vi "GV_StoreNewZoomValue.vi"(7 "Immediate":bool, 8 "error in (no error)":errorcluster, 11 "Gviewer in":refnum<class "Gviewer.lvclass">) -> (0 "error out":errorcluster, 3 "Gviewer out":refnum<class "Gviewer.lvclass">)   [LabVIEW 2020, in "Sgraph_lib_V1.lvlib" / "Gviewer.lvclass"]
doc: "Set the new pan or zoom value to the undo memory"
uses:
  Gviewer.lvclass
  Gviewer.lvclass/Gviewer.ctl
  controls/Typedef_ZoomEvent.ctl
  controls/Typedef_Live.ctl
  controls/Typedef_SelProperties.ctl
  controls/Typedef_LineType.ctl
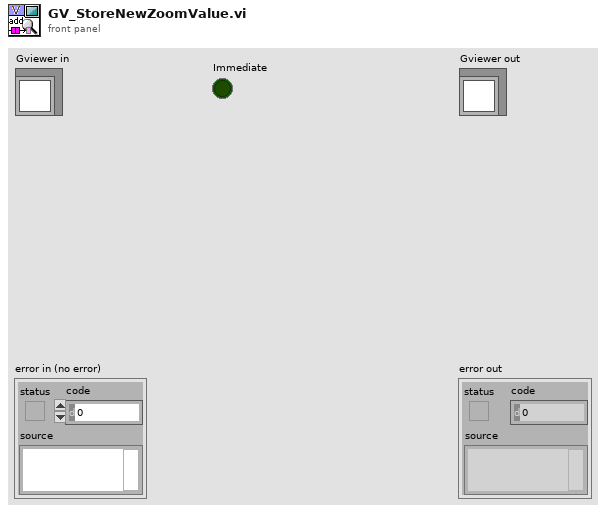
[diagram p1: front panel]
types:
  T1 = typedef "Sgraph_lib_V1.lvlib/Gviewer.lvclass/Typedef_ZoomEvent.ctl" = cluster{"Time-Start":timestamp, "Time-End":timestamp, "TimeSpan(sec)":dbl, "Live":T2, "SelProperties":T3[], "Time Stamp":timestamp}
  T2 = typedef "Sgraph_lib_V1.lvlib/Gviewer.lvclass/Typedef_Live.ctl" = enum16{"Live View", "Freeze"}
  T3 = typedef "Sgraph_lib_V1.lvlib/Gviewer.lvclass/Typedef_SelProperties.ctl" = cluster{"Color":u32, "LineType":T4, "max":dbl, "min":dbl}
  T4 = typedef "Sgraph_lib_V1.lvlib/Gviewer.lvclass/Typedef_LineType.ctl" = enum16{"num_bare", "num_MinMax_Area", "num_MinMax_Lines", "num_MinMax_Forfor", "num_Max_Area", "num_Max_Line", "num_Max_Forfor", "num_Min_Area", "num_Min_Line", "num_Min_Fosfor", "Boolean_Line_01", "Boolean_Area_01", "Boolean_Fosfor_01", "Boolean_Line_TF", "Boolean_Area_TF", "Boolean_Fosfor_TF", "Boolean_OnOff_Line", "Boolean_OnOff_Area", "Boolean_OnOff_Fosfor", "Boolean_spare", "StringEvent_Line", "StringEvent_TimeLine"}
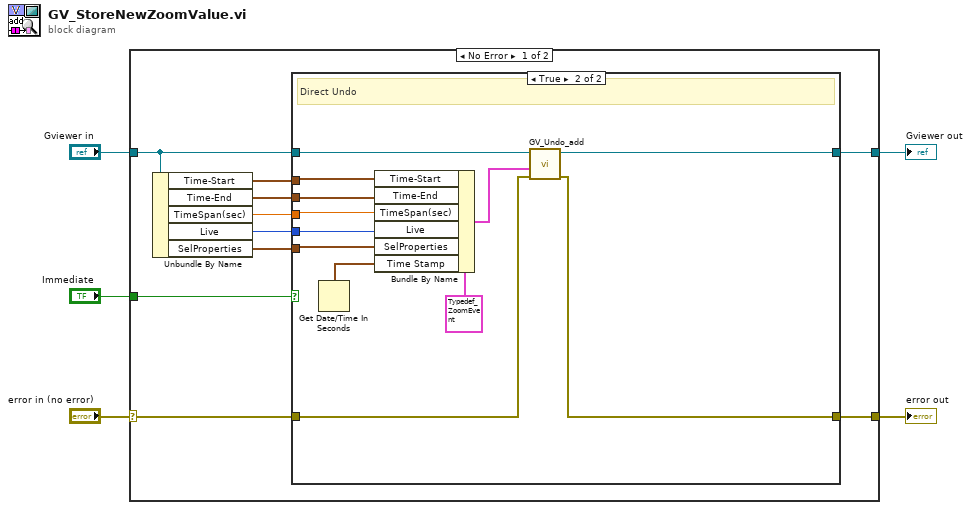
[diagram p0: block diagram]
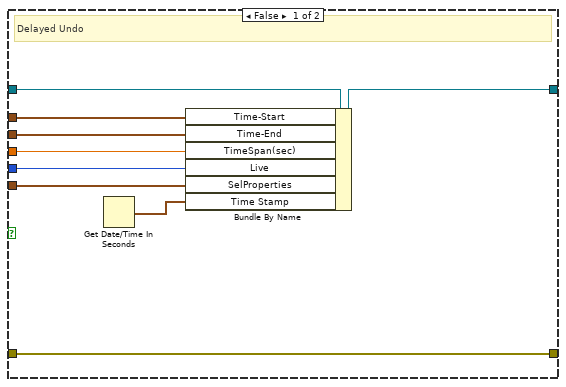
[diagram p2: hidden frame]
diagram:
  n1 = case shown="No Error" "error in (no error)" {
    selector: "error in (no error)" -> [w8 w38]
    tunnel: [w6 w38] -> w4
    tunnel: [w7 w37] -> w2
    tunnel: "Gviewer in" -> [w9 w37]
    tunnel: "Immediate" -> [w15 _]
    frame No Error {
      n2 = Unbundle By Name(w9) -> ("Time-Start"=w14:timestamp, "Time-End"=w13:timestamp, "TimeSpan(sec)"=w12:dbl, "Live"=w11:T2, "SelProperties"=w10:T3[])
      n3 = case shown="True" w15 {
        tunnel: w14 -> [w23 w31]
        tunnel: w13 -> [w22 w30]
        tunnel: w12 -> [w21 w29]
        tunnel: w11 -> [w20 w28]
        tunnel: w10 -> [w19 w27]
        tunnel: w9 -> [w16 w35]
        tunnel: w8 -> [w24 w33]
        tunnel: [w17 w36] -> w7
        tunnel: [w24 w34] -> w6
        frame False {
          # "Delayed Undo"
          n4 = Get Date/Time In Seconds() -> (seconds since 1Jan1904=w18:timestamp)
          n5 = Bundle By Name(cluster=w16, "Time-Start"=w23, "Time-End"=w22, "TimeSpan(sec)"=w21, "Live"=w20, "SelProperties"=w19, "Time Stamp"=w18) -> (w17:refnum<class "Gviewer.lvclass">)
        }
        frame True {
          # "Direct Undo"
          n6 = Get Date/Time In Seconds() -> (seconds since 1Jan1904=w26:timestamp)
          n7 = Bundle By Name(cluster=T1 {"Time-Start"=timestamp(0 s since 1904-01-01), "Time-End"=timestamp(0 s since 1904-01-01), "TimeSpan(sec)"=0.0, "Live"=enum."Live View", "SelProperties"=[], "Time Stamp"=timestamp(0 s since 1904-01-01)} ("ZoomEvent"), "Time-Start"=w31, "Time-End"=w30, "TimeSpan(sec)"=w29, "Live"=w28, "SelProperties"=w27, "Time Stamp"=w26) -> (w25:T1)
          n8 = call "GV_Undo_add.vi"("error in (no error)"=w33, "ZoomEvent"=w25, "Gviewer in"=w35) -> ("error out"=w34:errorcluster, "Gviewer out"=w36:refnum<class "Gviewer.lvclass">)  [unwired: 7 in]
        }
      }
    }
    frame Error {
    }
  }
  "error out" <- w4
  "Gviewer out" <- w2
